vi "rqcBob Mod Level Test - 2 SPD (Low Level Example).vi"() -> ()   [LabVIEW 2018]
uses:
  FPGA/rqcBob/Custom Controls/Pulse Train/rqcBob Pulse Train Config.ctl
  FPGA/rqcBob/Custom Controls/Pulse Train/rqcBob Pulse Train.Generation Mode.ctl
  FPGA/rqcBob/Custom Controls/Pulse Train/rqcBob Pulse Train.First Pulse Delay Mode.ctl
  FPGA/rqcBob/Custom Controls/rqcBob Modulator Config.ctl
  FPGA/rqcBob/Custom Controls/rqcBob Window Config.ctl
  Shared/Shared FPGA Lib/Shared Logic/Custom Controls/rqc Random Generator.parameters.ctl
  Shared/Shared FPGA Lib/Shared Logic/Custom Controls/rqc Random Generator.value type.ctl
  FPGA/rqcBob/Custom Controls/rqcBob Trigger Type.ctl
  <vilib>/Analysis/1siggen.llb/Ramp Pattern by Delta.vi
  <vilib>/FPGAPlugInAG/PCIe-7820R/niLvFpga_Open_PCIe-7820R.vi
  <vilib>/rvi/interface/common/dynamic/niFpgaDynamicAddResources.vi
  Low Level API/Configuration/Photon Detector/Detection FIFOs config/rqcBob Configure PD Detect FIFO (1PD PD1).vi
  Low Level API/Read/Read PD Detection FIFO/rqcBob Read PD Detection FIFO (1PD PD1).vi
  <vilib>/FPGAPlugInAG/Dynamic/niLvFpga_Close_Dynamic.vi
  <vilib>/rvi/interface/nirviOpenFPGA/nirviOpenFPGA.xnode
  FPGA Bitfiles/rqcBob (FPGA) 7820 v 2.1.1.lvbitx
  <vilib>/rvi/interface/nirviCloseFPGA/nirviCloseFPGA.xnode
  <vilib>/Analysis/NI_AALBase.lvlib
panel:
  in  "modulator.clock delay":fxp<+,4,4>
  out "Progress":dbl(slide)=32.30769230769231 scale=0.0..100.0
  out "Num of Detections vs DAC Level":cluster{u16[], "appended array":dbl[]}(graph)={[0, 8, 16, 24, 32, 40, 48, 56, 64, 72, 80, 88, 96, 104, 112, 120, 128, 136, 144, 152, 160, 168, 176, 184, 192, 200, 208, 216, 224, 232, 240, 248, 256, 264, 272, 280, 288, 296, 304, 312, 320, 328, 336, 344, 352, 360, 368, 376, 384, 392, 400, 408, 416, 424, 432, 440, 448, 456, 464, 472, 480, 488, 496, 504, 512], "appended array"=[7097.0, 7109.0, 6146.0, 6152.0, 7113.0, 6205.0, 6199.0, 6219.0, 6236.0, 6185.0, 6222.0, 7085.0, 6242.0, 7123.0, 6279.0, 6196.0, 6245.0, 6247.0, 6220.0, 6194.0, 5346.0]}
  in  "stop":bool
  in  "DAC interval":u16=8
  in  "DAC Level max":u16=512
  in  "DAC Level min":u16
  in  "rndGen.parameters":T1={"value type"=enum."constant", "constant"=0, "num of levels"=0, "levels values"=[0, 0, 0, 0]}
  in  "window.config":T3={"window.open"=1340, "window.close"=300}
  in  "modulator.config":T4={"modulator.start"=1000, "modulator.stop"=2700}
  in  "train.configuration":T5={"period"=2200, "num of pulses"=300, "mode"=enum."train sequence.single", "num of trains"=1000, "first pulse delay mode"=enum."every train", "first pulse delay"=55}
  out "Done":bool
  # "PM Level Settings"
  # "Bob configuration"
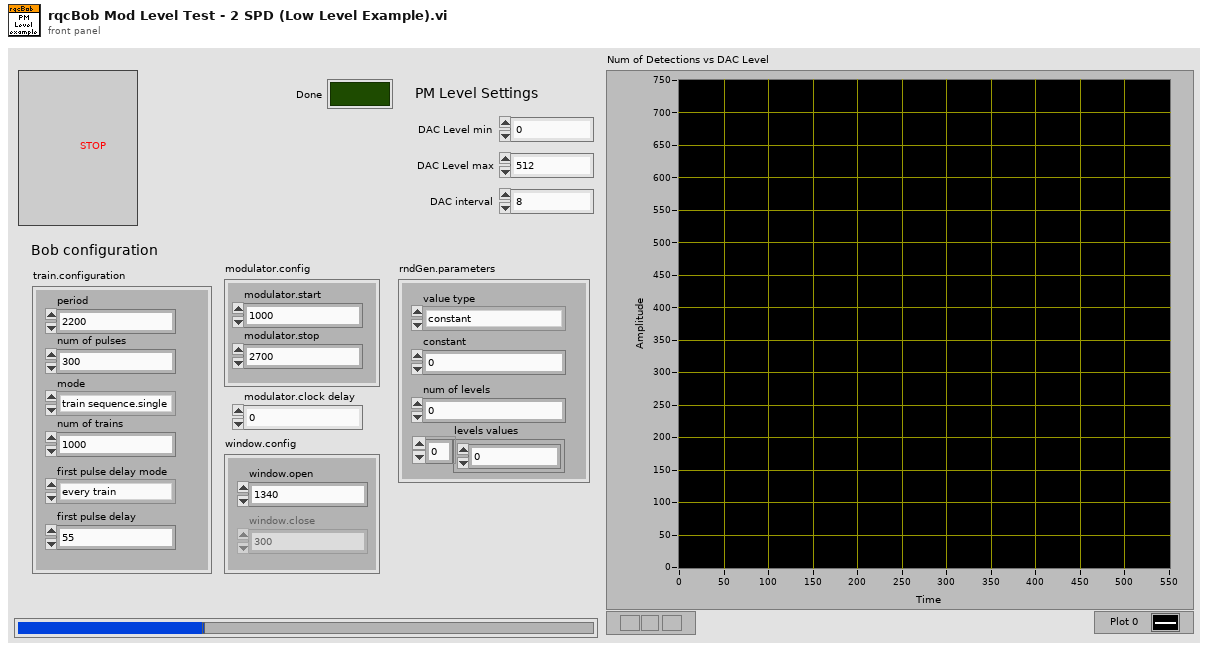
[diagram p1: front panel]
types:
  T1 = typedef "rqc Random Generator.parameters.ctl" = cluster{"value type":T2, "constant":u16, "num of levels":u16, "levels values":u16[]}
  T2 = typedef "rqc Random Generator.value type.ctl" = enum16{"random value", "constant"}
  T3 = typedef "rqcBob Window Config.ctl" = cluster{"window.open":u16, "window.close":u16}
  T4 = typedef "rqcBob Modulator Config.ctl" = cluster{"modulator.start":u16, "modulator.stop":u16}
  T5 = typedef "rqcBob Pulse Train Config.ctl" = cluster{"period":u16, "num of pulses":u16, "mode":T6, "num of trains":u16, "first pulse delay mode":T7, "first pulse delay":u16}
  T6 = typedef "rqcBob Pulse Train.Generation Mode.ctl" = enum8{"single train", "train sequence.single", "train sequence.wait for trigger", "continuous"}
  T7 = typedef "rqcBob Pulse Train.First Pulse Delay Mode.ctl" = enum8{"none", "every train", "first train"}
  T8 = typedef "rqcBob Trigger Type.ctl" = enum16{"software", "immediate", "DIO"}
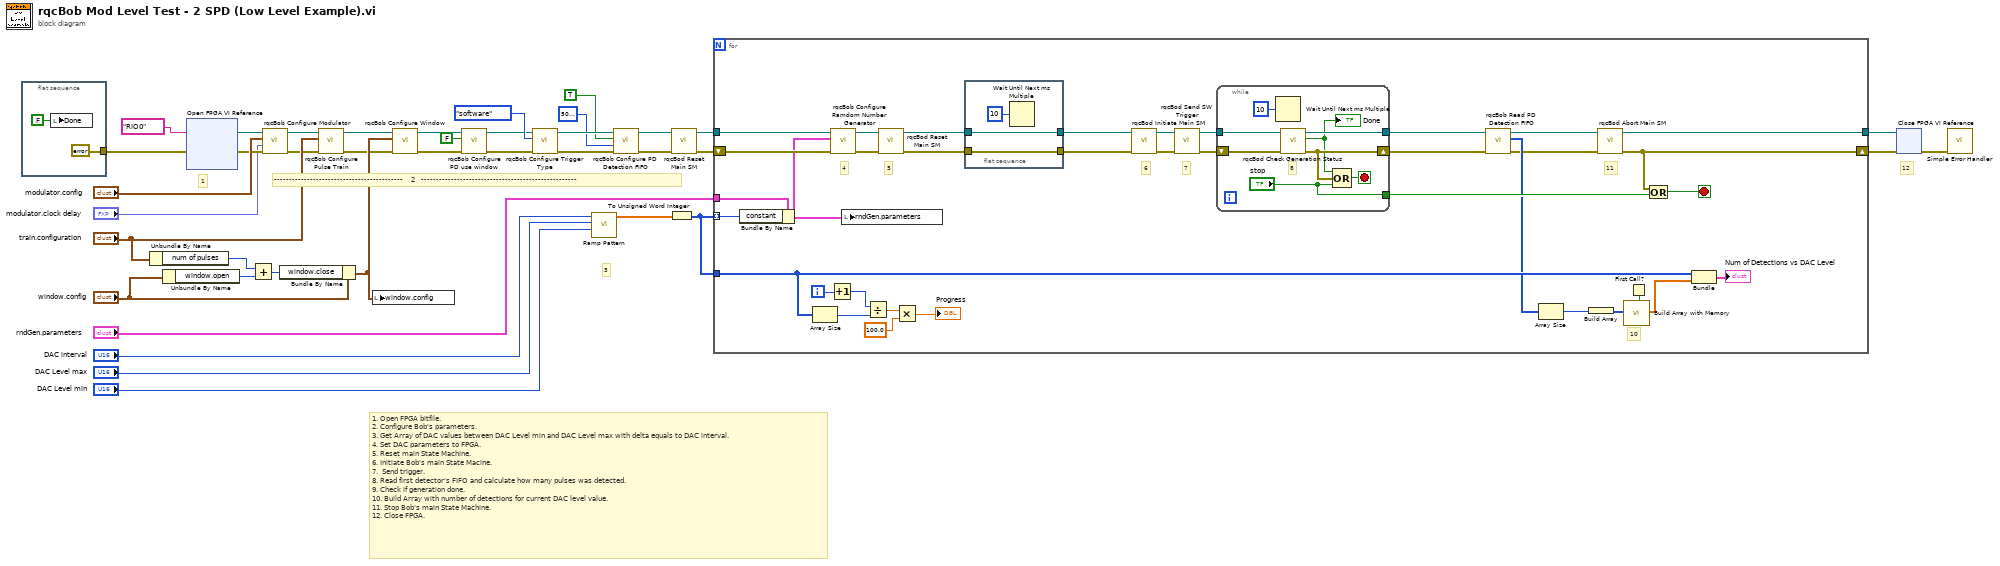
[diagram p0: block diagram]
diagram:
  # "12"
  # "3"
  # "1. Open FPGA bitfile.\n2. Configure Bob's parameters.\n3. Get Array of DAC values between DAC Level min and DAC Level max with delta equals to DAC interval.\n4. Set DAC parameters to FPGA.\n5. Reset main State Machine.\n6. Initiate Bob's main State Macine.\n7.  Send trigger.\n8. Read first detector's FIFO and calculate how many pulses was detected.\n9. Check if generation done.\n10. Build Array with number of detections for current DAC level value.\n11. Stop Bob's main State Machine.\n12. Close FPGA."
  # "1"
  # "-------------------------------------------    2   ----------------------------------------------------"
  n1 = flat-sequence {
    tunnel: [errorcluster {"status"=FALSE, "code"=0, "source"=""} ("error in")] -> w36
    frame #0 {
      n2 = local write "Done"(FALSE ("Done")) -> ()
    }
  }
  n3 = Unbundle By Name("train.configuration") -> ("num of pulses"=w34:u16)
  n4 = Unbundle By Name("window.config") -> ("window.open"=w33:u16)
  n5 = xnode "Open FPGA VI Reference"("error in"=w36, "resource name"=tag "RIO0") -> ("FPGA VI Reference Out"=w11:refnum<k20>, "error out"=w10:errorcluster)
  n6 = Add(x=w34, y=w33) -> (x+y=w31:u16)
  n7 = call "rqcBob Configure Modulator.vi"("error in"=w10, "modulator.clock delay"="modulator.clock delay", "modulator.config"="modulator.config", "FPGA reference in"=w11) -> ("error out"=w24:errorcluster, "FPGA reference out"=w25:refnum<k20>)  [unwired: 6 in]
  n8 = Bundle By Name(cluster="window.config", "window.close"=w31) -> (w30:T3)
  n9 = call "rqcBob Configure Pulse Train.vi"("error in"=w24, "train.configuration"="train.configuration", "FPGA reference in"=w25) -> ("error out"=w26:errorcluster, "FPGA reference out"=w27:refnum<k20>)  [unwired: 6 in, 1 out]
  n10 = local write "window.config"(w30) -> ()
  n11 = call "rqcBob Configure Window.vi"("error in"=w26, "window.config"=w30, "FPGA reference in"=w27) -> ("error out"=w28:errorcluster, "FPGA reference out"=w29:refnum<k20>)  [unwired: 7 in]
  n12 = call "rqcBob Configure PD use window.vi"("error in"=w28, "PD.use window"=FALSE ("SPD.use detector window"), "FPGA reference in"=w29) -> ("error out"=w1:errorcluster, "FPGA reference out"=w2:refnum<k20>)  [unwired: 7 in]
  n13 = call "rqcBob Configure Trigger Type.vi"("error in"=w1, "rqcBob Trigger Type"=rqcBob_Trigger_Type."software", "FPGA reference in"=w2) -> ("error out"=w6:errorcluster, "FPGA reference out"=w8:refnum<k20>)  [unwired: 7 in]
  n14 = call-poly <vilib>:"Ramp Pattern.vi"("start"="DAC Level min", "end"="DAC Level max", "delta"="DAC interval") -> ("Ramp Pattern"=w20:dbl[])  [unwired: 6 in, 2 out]
  n15 = call-poly "rqcBob Configure PD Detection FIFO.vi"("error in"=w6, "PD.detect fifo depth"=u32 5000000 ("SPD.detect fifo depth"), "PD.detect fifo write enable"=TRUE ("SPD.detect fifo write enable"), "FPGA reference in"=w8) -> ("error out"=w3:errorcluster, "FPGA reference out"=w7:refnum<k20>)  [unwired: 6 in]
  n16 = To Unsigned Word Integer(number=w20) -> (unsigned 16bit integer=w19:u16[])
  n17 = call "rqcBod Reset Main SM.vi"("error in"=w3, "FPGA reference in"=w7) -> ("error out"=w13:errorcluster, "FPGA reference out"=w14:refnum<k20>)  [unwired: 8 in]
  n18 = for {
    tunnel: w14 -> [w75]
    tunnel: w19 -> [w47] mode=indexing
    tunnel: "rndGen.parameters" -> [w73]
    tunnel: [w70] -> w18
    shift-right: [w68] -> w17
    shift-left: w13 -> [w74]
    tunnel: w19 -> [w56]
    i -> [w57]
    stop <- w66 stop-if-true
    # "5"
    # "11"
    # "10"
    # "7"
    # "6"
    # "4"
    n19 = Bundle By Name(cluster=w73, "constant"=w47) -> (w67:T1)
    n20 = Array Size(array=w56) -> (size(s)=w65:i32)
    n21 = Increment(x=w57) -> (x+1=w64:i32)
    n22 = call "rqcBob Configure Ramdom Number Generator.vi"("error in"=w74, "rqcBob rndGen.parameters"=w67, "FPGA reference in"=w75) -> ("error out"=w52:errorcluster, "FPGA reference out"=w53:refnum<k20>)  [unwired: 7 in]
    n23 = local write "rndGen.parameters"(w67) -> ()
    n24 = Divide(x=w64, y=w65) -> (x/y=w63:dbl)
    n25 = call "rqcBod Reset Main SM.vi"("error in"=w52, "FPGA reference in"=w53) -> ("error out"=w48:errorcluster, "FPGA reference out"=w49:refnum<k20>)  [unwired: 8 in]
    n26 = Multiply(x=w63, y=100.0) -> (x*y=→"Progress":dbl)
    n27 = flat-sequence {
      tunnel: [w80] -> w51
      tunnel: w49 -> [w80]
      tunnel: [w79] -> w50
      tunnel: w48 -> [w79]
      frame #0 {
        n28 = Wait Until Next ms Multiple(millisecond multiple=u32 10) -> ()  [unwired: 1 out]
      }
    }
    n29 = call "rqcBod Initiate Main SM.vi"("error in"=w50, "FPGA reference in"=w51) -> ("error out"=w76:errorcluster, "FPGA reference out"=w77:refnum<k20>)  [unwired: 8 in]
    n30 = call "rqcBod Send SW Trigger.vi"("error in"=w76, "FPGA reference in"=w77) -> ("error out"=w71:errorcluster, "FPGA reference out"=w72:refnum<k20>)  [unwired: 8 in]
    n31 = while {
      tunnel: w72 -> [w83]
      shift-right: [w88] -> w44
      shift-left: w71 -> [w84]
      tunnel: [w82] -> w46
      tunnel: ["stop"] -> w69
      stop <- w87 stop-if-true
      # "8"
      n32 = Wait Until Next ms Multiple(millisecond multiple=u32 10) -> ()  [unwired: 1 out]
      n33 = call "rqcBod Check Generation Status.vi"("error in"=w84, "FPGA reference in"=w83) -> ("error out"=w88:errorcluster, "generation.done"=w81:bool, "FPGA reference out"=w82:refnum<k20>)  [unwired: 7 in]
      "Done" <- w81
      n34 = Compound Arithmetic op=OR(w81, w88, "stop") -> (w87:bool)
    }
    n35 = call-poly "rqcBob Read PD Detection FIFO.vi"("error in"=w44, "FPGA reference in"=w46) -> ("error out"=w42:errorcluster, "Data"=w43:u32[], "FPGA reference out"=w45:refnum<k20>)  [unwired: 6 in, 1 out]
    n36 = Array Size(array=w43) -> (size(s)=w54:i32)
    n37 = Build Array(w54) -> (w59:i32[])
    n38 = call "rqcBod Abort Main SM.vi"("error in"=w42, "FPGA reference in"=w45) -> ("error out"=w68:errorcluster, "FPGA reference out"=w70:refnum<k20>)  [unwired: 8 in]
    n39 = First Call?() -> (First Call?: T/F=w58:bool)
    n40 = call "Build Array with Memory.vi"("reset"=w58, "new array"=w59) -> ("appended array"=w60:dbl[])  [unwired: 9 in]
    n41 = Compound Arithmetic op=OR(w68, w69) -> (w66:bool)
    n42 = Bundle(w56, "appended array"=w60) -> (→"Num of Detections vs DAC Level":cluster{u16[], "appended array":dbl[]})  [unwired: 1 in]
  }
  n43 = xnode "Close FPGA VI Reference"("FPGA VI Reference In"=w18, "error in"=w17) -> ("error out"=w16:errorcluster)
  n44 = call <vilib>:"Simple Error Handler.vi"("error in (no error)"=w16) -> ()  [unwired: 4 in, 5 out]
